vi "Connect.vi"(8 "error in (no error)":errorcluster, 10 "Instrument Index":i32, 11 "PalmSens in":refnum<class "PalmSens.lvclass">) -> (0 "error out":errorcluster, 3 "PalmSens out":refnum<class "PalmSens.lvclass">)   [LabVIEW 2025, in "PalmSens.lvclass"]
uses:
  PalmSens.lvclass
  PalmSens.lvclass/PalmSens.ctl
  E:/PSCode/PalmSens_SDK/labview/PalmSens/Libraries/PalmSens.Core.Simplified.LabVIEW.dll
  Libraries/PalmSens.Core.Simplified.LabVIEW.dll
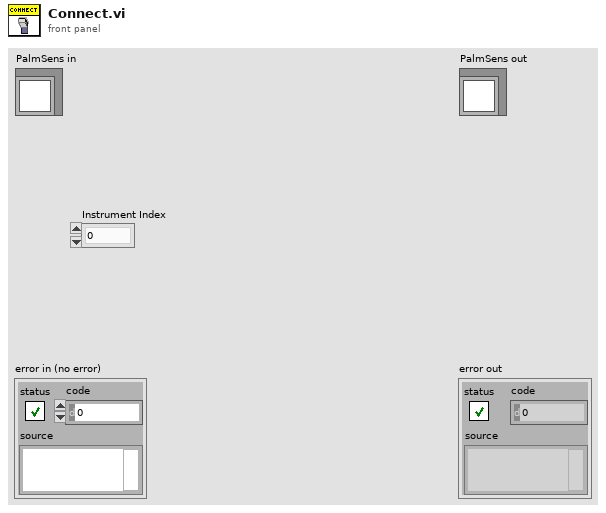
[diagram p1: front panel]
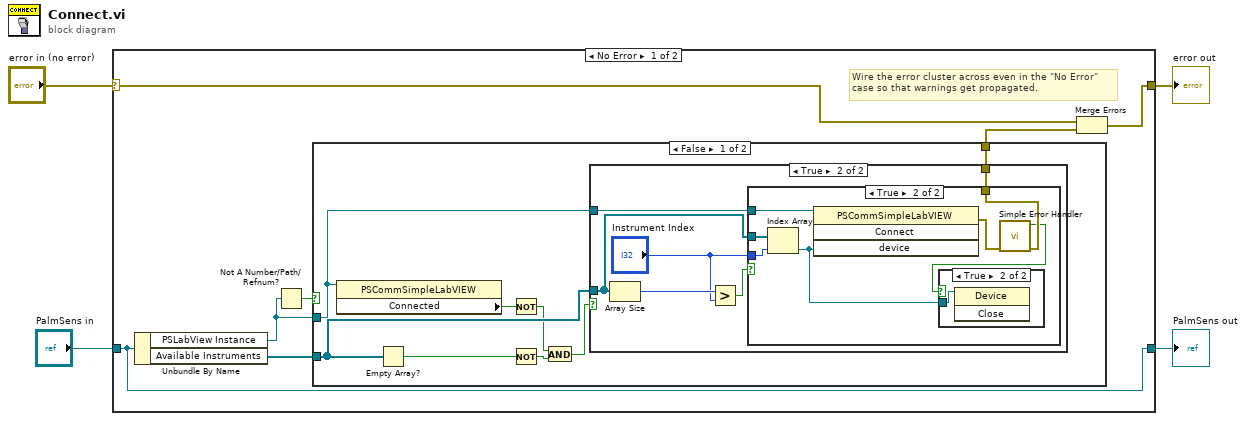
[diagram p0: block diagram]
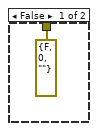
[diagram p2: hidden frame]
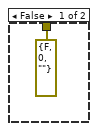
[diagram p3: hidden frame]
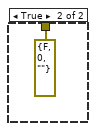
[diagram p5: hidden frame]
diagram:
  n1 = case shown="No Error" "error in (no error)" {
    selector: "error in (no error)" -> [w6 w38]
    tunnel: [w5 w38] -> w3
    tunnel: [w11 w37] -> w1
    tunnel: "PalmSens in" -> [w11 w37]
    frame No Error {
      # "Wire the error cluster across even in the \"No Error\"\ncase so that warnings get propagated."
      n2 = Unbundle By Name(w11) -> ("PSLabView Instance"=w9:refnum<k24>, "Available Instruments"=w8:refnum<k24>[])
      n3 = Not A Number/Path/Refnum?(number/path/refnum=w9) -> (NaN/Path/Refnum?=w10:bool)
      n4 = case shown="False" w10 {
        tunnel: w9 -> [w18 _]
        tunnel: w8 -> [w19 _]
        tunnel: [w12 errorcluster {"status"=FALSE, "code"=0, "source"=""} ("error out")] -> w7
        frame False {
          n5 = property class="PSCommSimpleLabVIEW"(reference=w18) -> ("Connected"=w15:bool)  [unwired: 1 in, 2 out]
          n6 = Empty Array?(array=w19) -> (empty?=w17:bool)
          n7 = Not(x=w15) -> (.not. x?=w14:bool)
          n8 = Not(x=w17) -> (.not. x?=w16:bool)
          n9 = And(x=w14, y=w16) -> (x .and. y?=w13:bool)
          n10 = case shown="True" w13 {
            tunnel: w18 -> [_ w26]
            tunnel: w19 -> [_ w23]
            tunnel: [errorcluster {"status"=FALSE, "code"=0, "source"=""} ("error out") w21] -> w12
            frame False {
            }
            frame True {
              n11 = Array Size(array=w23) -> (size(s)=w25:i32)
              n12 = Greater?(x=w25, y="Instrument Index") -> (0:w24:bool)
              n13 = case shown="True" w24 {
                tunnel: w26 -> [_ w34]
                tunnel: w23 -> [_ w33]
                tunnel: "Instrument Index" -> [_ w32]
                tunnel: [errorcluster {"status"=FALSE, "code"=0, "source"=""} ("error out") w30] -> w21
                frame False {
                }
                frame True {
                  n14 = Index Array(array=w33, index=w32) -> (element=w28:refnum<k24>)
                  n15 = invoke class="PSCommSimpleLabVIEW" method="Connect"(reference=w34, "device"=w28) -> (error out=w31:errorcluster)  [unwired: 2 in, 3 out]
                  n16 = call <vilib>:"Simple Error Handler.vi"("error in (no error)"=w31) -> ("error?"=w29:bool, "error out"=w30:errorcluster)  [unwired: 4 in, 3 out]
                  n17 = case shown="True" w29 {
                    tunnel: w28 -> [_ w35]
                    frame False {
                    }
                    frame True {
                      n18 = invoke class="Device" method="Close"(reference=w35) -> ()  [unwired: 2 in, 3 out]
                    }
                  }
                }
              }
            }
          }
        }
        frame True {
        }
      }
      n19 = Merge Errors(w6, w7) -> (w5:errorcluster)
    }
    frame Error {
    }
  }
  "error out" <- w3
  "PalmSens out" <- w1
